vi "e.gate HighSpeedPort Online Communication - CORE.vi"(0 "WriteIndex":i32, 1 "WriteCount":i32, 2 "ValueArray":dbl[](array[numeric]), 3 "ReadIndex":i32, 4 "ReadCount":i32, 7 "error in (no error)":errorcluster, 8 "Configuration in":T1) -> (18 "Configuration out":T1, 21 "data array (binary)":u8[](array[numeric]), 27 "error out":errorcluster)   [LabVIEW 2016]
doc: "This VI is used to perform HighSpeedPort TCP/IP online communication between Gantner Instruments e.series controller and LabView."
uses:
  e.gate Configuration.ctl
  e.gate Channel Data.ctl
  e.gate Data Type.ctl
  e.gate Protocol Type.ctl
  e.gate Module  Data.ctl
  e.gateHSP_DLLhandle.ctl
panel:
  out "DataWrite":string
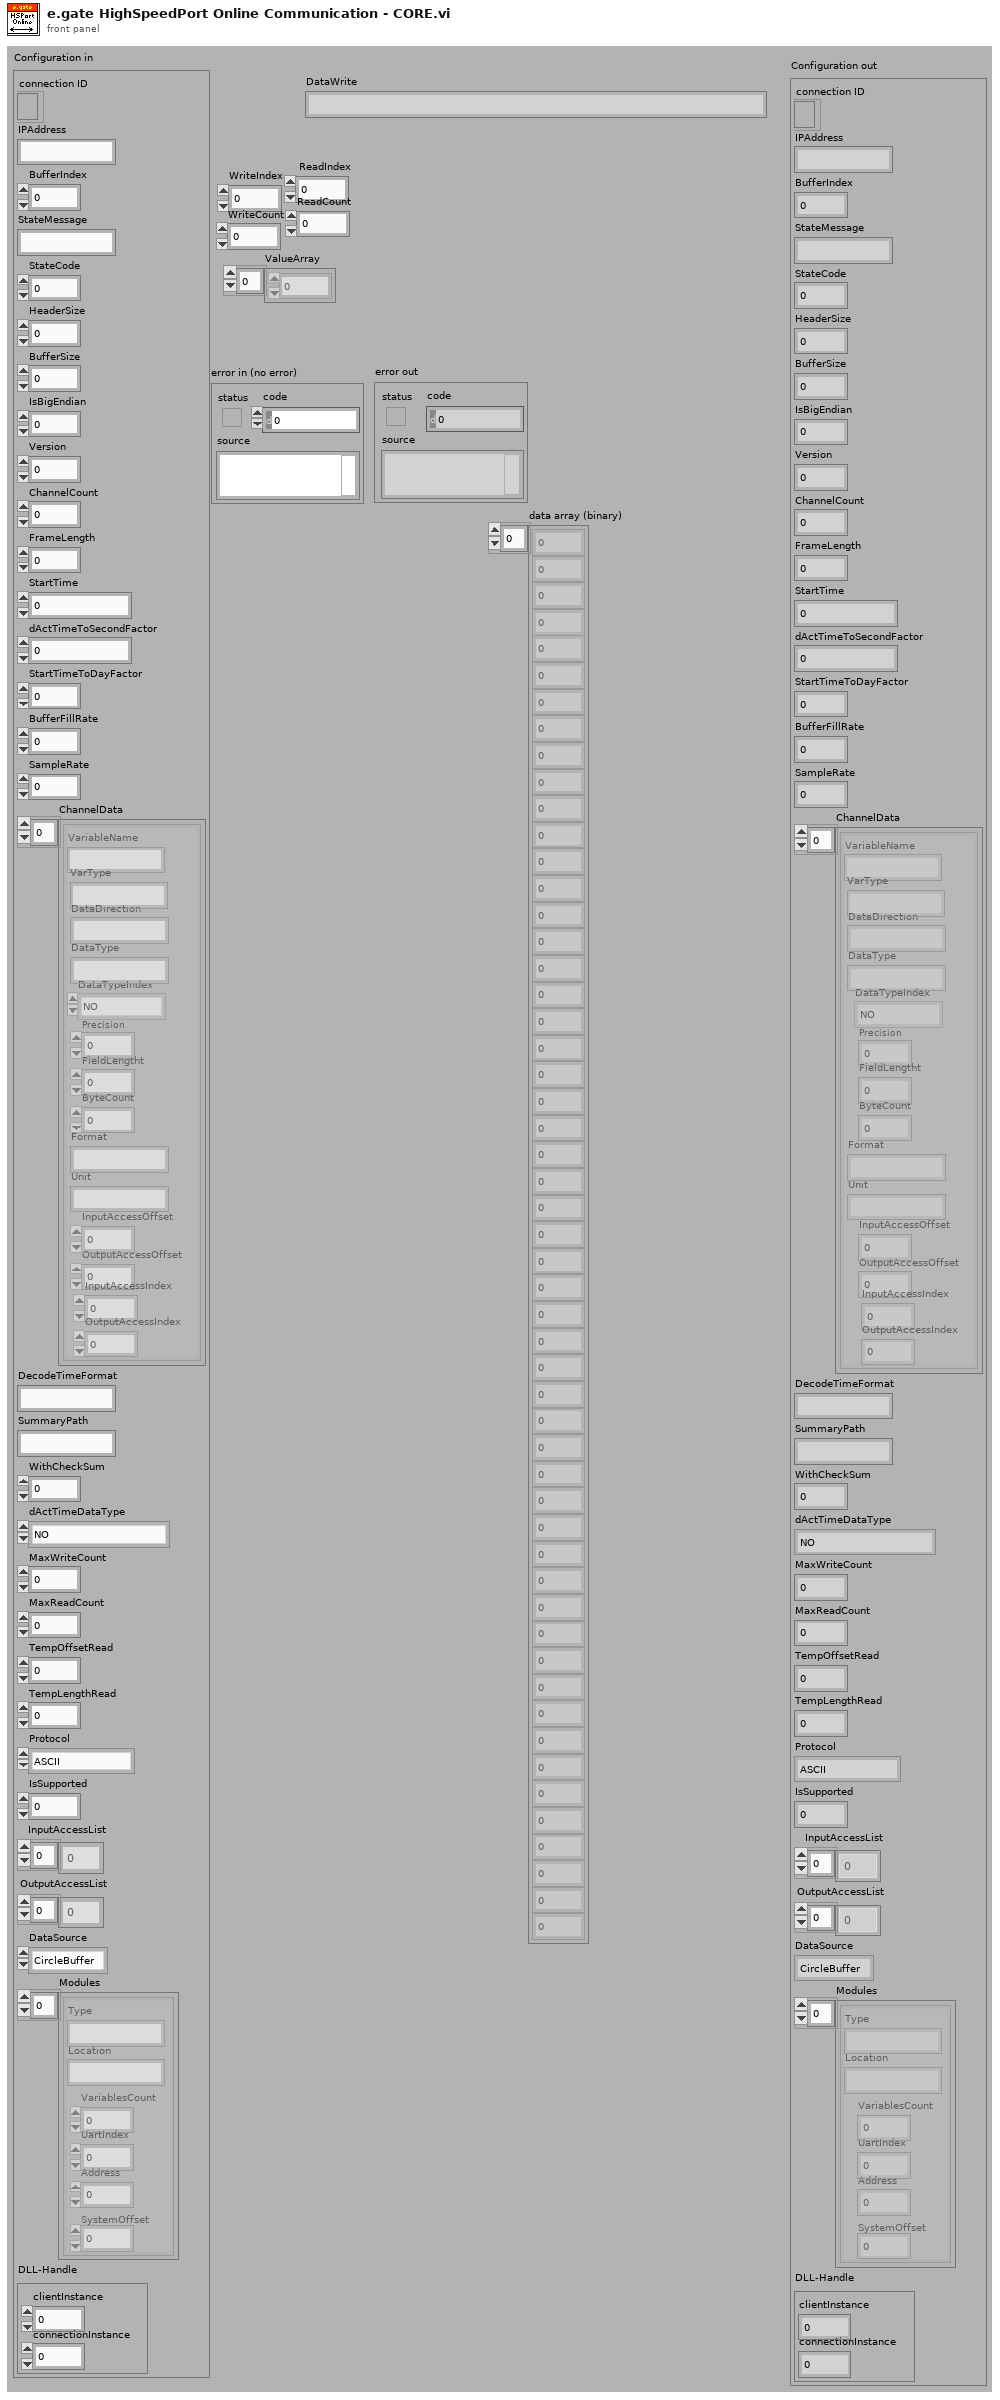
[diagram p1: front panel]
types:
  T1 = typedef "e.gate Configuration.ctl" = cluster{"connection ID":refnum<k5>, "IPAddress":string, "BufferIndex":i32, "StateMessage":string, "StateCode":i8, "HeaderSize":i32, "BufferSize":i32, "IsBigEndian":i32, "Version":i32, "ChannelCount":i32, "FrameLength":i32, "StartTime":dbl, "dActTimeToSecondFactor":dbl, "StartTimeToDayFactor":dbl, "BufferFillRate":dbl, "SampleRate":dbl, "ChannelData":T2[], "DecodeTimeFormat":string, "SummaryPath":string, "WithCheckSum":i32, "dActTimeDataType":T3, "MaxWriteCount":i32, "MaxReadCount":i32, "TempOffsetRead":i32, "TempLengthRead":i32, "Protocol":T4, "IsSupported":i32, "InputAccessList":i32[], "OutputAccessList":i32[], "DataSource":enum16{"CircleBuffer", "test.con Logger", "test.con Archive"}, "Modules":T5[], "DLL-Handle":T6}
  T2 = typedef "e.gate Channel Data.ctl" = cluster{"VariableName":string, "DataDirection":string, "DataType":string, "DataTypeIndex":T3, "Precision":i16, "FieldLengtht":i16, "ByteCount":i32, "Format":string, "Unit":string, "InputAccessOffset":i32, "OutputAccessOffset":i16, "InputAccessIndex":i16, "OutputAccessIndex":i16, "VarType":string}
  T3 = typedef "e.gate Data Type.ctl" = enum16{"NO", "BOOL", "SINT8", "USINT8", "SINT16", "USINT16", "SINT32", "USINT32", "FLOAT", "SET8", "SET16", "SET32", "DOUBLE", "SINT64", "USINT64", "SET64"}
  T4 = typedef "e.gate Protocol Type.ctl" = enum16{"ASCII", "HighspeedPort Online", "HighspeedPort Buffer", "eGateHighspeedPortDLL "}
  T5 = typedef "e.gate Module  Data.ctl" = cluster{"Type":string, "Location":string, "VariablesCount":i16, "UartIndex":i16, "Address":i16, "SystemOffset":i16}
  T6 = typedef "e.gateHSP_DLLhandle.ctl" = cluster{"clientInstance":i32, "connectionInstance":i32}
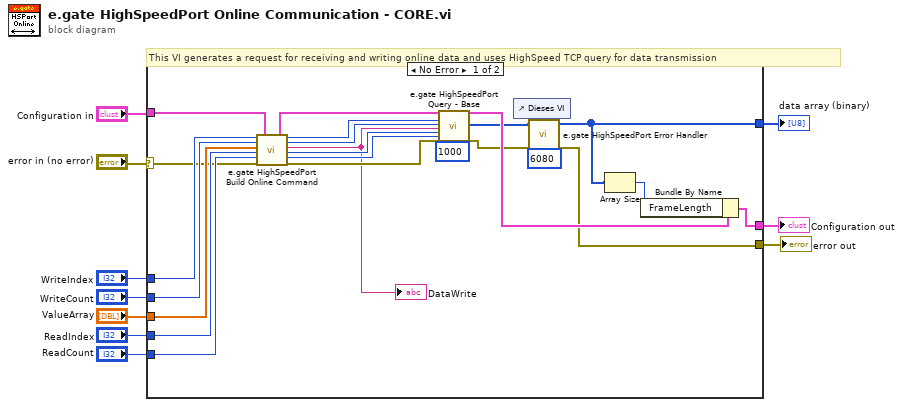
[diagram p0: block diagram]
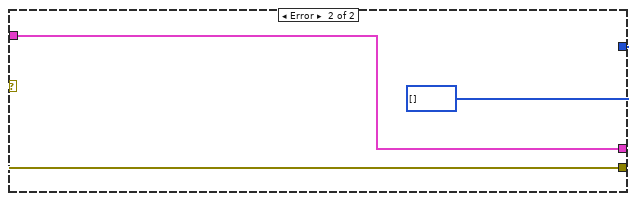
[diagram p2: hidden frame]
diagram:
  # "This VI generates a request for receiving and writing online data and uses HighSpeed TCP query for data transmission"
  n1 = case shown="No Error" "error in (no error)" {
    selector: "error in (no error)" -> [w20 w37]
    tunnel: [w11 u8[] [] ("unsigned byte array")] -> w10
    tunnel: [w12 w37] -> w1
    tunnel: "Configuration in" -> [w33 w35]
    tunnel: [w26 w35] -> w4
    tunnel: "WriteIndex" -> [w31 _]
    tunnel: "WriteCount" -> [w30 _]
    tunnel: "ValueArray" -> [w29 _]
    tunnel: "ReadIndex" -> [w28 _]
    tunnel: "ReadCount" -> [w27 _]
    frame No Error {
      n2 = call "e.gate HighSpeedPort Build Online Command.vi"("WriteIndex"=w31, "WriteCount"=w30, "ValueArray"=w29, "ReadIndex"=w28, "ReadCount"=w27, "error in (no error)"=w20, "Configuration  in"=w33) -> ("Configuration  out"=w19:T1, "OffsetWrite"=w21:i32, "LengthWrite"=w22:i32, "DataWrite"=w23:string, "OffsetRead"=w24:i32, "LengthRead"=w25:i32, "error out"=w32:errorcluster)  [unwired: 6 out]
      "DataWrite" <- w23
      n3 = call "e.gate HighSpeedPort Query - Base.vi"("e.gate Configuration in"=w19, "OffsetWrite"=w21, "LengthWrite"=w22, "DataWrite"=w23, "OffsetRead"=w24, "LengthRead"=w25, "error in (no error)"=w32, "Timeout (1000)"=1000) -> ("e.gate Configuration out"=w18:T1, "Data (out binary)"=w14:u8[], "error out"=w13:errorcluster)  [unwired: 2 in, 15 out]
      n4 = control-ref of="Dieses VI"() -> (w16:refnum<vi>)
      n5 = call "e.gate HighSpeedPort Error Handler.vi"("error code start index"=6080, "VI reference"=w16, "error in (no error)"=w13, "binary data in"=w14) -> ("error out"=w12:errorcluster, "binary out"=w11:u8[])  [unwired: 6 out]
      n6 = Array Size(array=w11) -> (size(s)=w15:i32)
      n7 = Bundle By Name(cluster=w18, "FrameLength"=w15) -> (w26:T1)
    }
    frame Error {
    }
  }
  "data array (binary)" <- w10
  "Configuration out" <- w4
  "error out" <- w1
